vi "Create Sample Offset DVR.vi"(8 "error in (no error)":errorcluster, 11 "Waveform Session in":refnum<class "Waveform Session.lvclass">) -> (0 "error out":errorcluster, 3 "Waveform Session out":refnum<class "Waveform Session.lvclass">)   [LabVIEW 2020, in "NI_VS Custom Device Waveform API.lvlib" / "Waveform Session.lvclass"]
uses:
  Waveform Session.lvclass
  Waveform Session.lvclass/Waveform Session.ctl
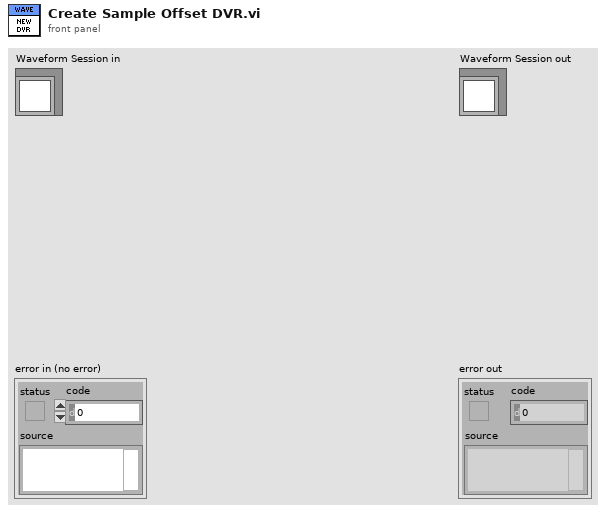
[diagram p1: front panel]
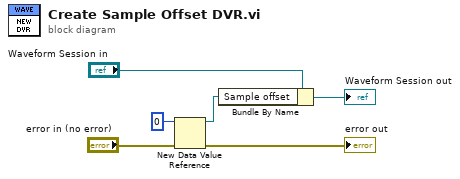
[diagram p0: block diagram]
diagram:
  n1 = New Data Value Reference(data value=u64 0, error in="error in (no error)") -> (data value reference=w1:refnum<data-value>, error out=→"error out":errorcluster)
  n2 = Bundle By Name(cluster="Waveform Session in", "Sample offset"=w1) -> (→"Waveform Session out":refnum<class "Waveform Session.lvclass">)
